vi "Parse Date.vi"(7 "Time In":T1, 10 "Date Index":i32, 11 "Fields In":string[](array[string])) -> (3 "Fields":string[](array[string]), 5 "Time":T1)   [LabVIEW 2012, in "nmea.lvlib" / "nmea.lvclass"]
uses:
  nmea.lvclass
  <vilib>/Utility/miscctls.llb/LVDateTimeRec.ctl
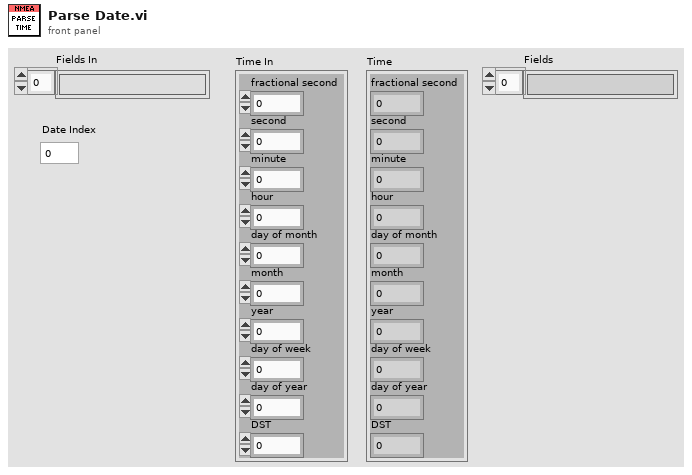
[diagram p1: front panel]
types:
  T1 = typedef "LVDateTimeRec.ctl" = cluster{"fractional second":dbl, "second":i32, "minute":i32, "hour":i32, "day of month":i32, "month":i32, "year":i32, "day of week":i32, "day of year":i32, "DST":i32}
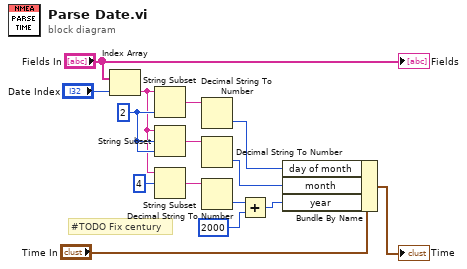
[diagram p0: block diagram]
diagram:
  w14 = 2 ("length (rest)")
  # "#TODO Fix century"
  n1 = Index Array(array="Fields In", index="Date Index") -> (element=w13:string)
  n2 = String Subset(string=w13, length (rest)=w14) -> (substring=w10:string)  [unwired: 1 in]
  n3 = String Subset(string=w13, offset (0)=w14, length (rest)=w14) -> (substring=w11:string)
  n4 = String Subset(string=w13, offset (0)=4) -> (substring=w4:string)  [unwired: 1 in]
  n5 = Decimal String To Number(string=w10) -> (number=w6:i32)  [unwired: 2 in, 1 out]
  n6 = Decimal String To Number(string=w11) -> (number=w7:i32)  [unwired: 2 in, 1 out]
  n7 = Decimal String To Number(string=w4) -> (number=w3:i32)  [unwired: 2 in, 1 out]
  n8 = Add(x=w3, y=2000) -> (x+y=w2:i32)
  n9 = Bundle By Name(cluster="Time In", "day of month"=w6, "month"=w7, "year"=w2) -> (→"Time":T1)
  "Fields" <- "Fields In"
